vi "REWORK_config_keys_to_cluster.vi"(8 "error_in":errorcluster, 9 "section_key_type_table":string[][](array[string]), 10 "reference_ini_file_path":path, 11 "config_cluster_ref":refnum<vi>) -> (0 "error_out":errorcluster, 3 "reference_info":T1)   [LabVIEW 2019]
uses:
  typedef/REWORK_config_info.ctl
  _misc/ini/config_info.ctl
  _misc/AULocalize/SubVIs/Get Localized Phrase Compact Interface 0D.vi
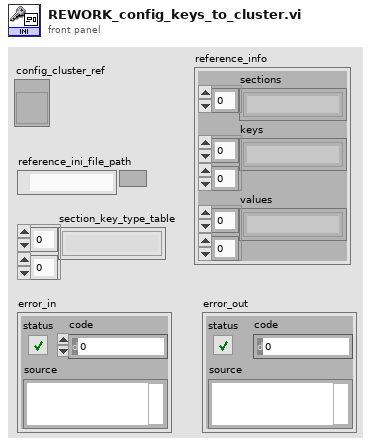
[diagram p1: front panel]
types:
  T1 = typedef "REWORK_config_info.ctl" = cluster{"sections":string[], "keys":string[][], "values":string[][]}
  T2 = typedef "config_info.ctl" = cluster{"sections":string[], "keys":string[][], "values":string[][]}
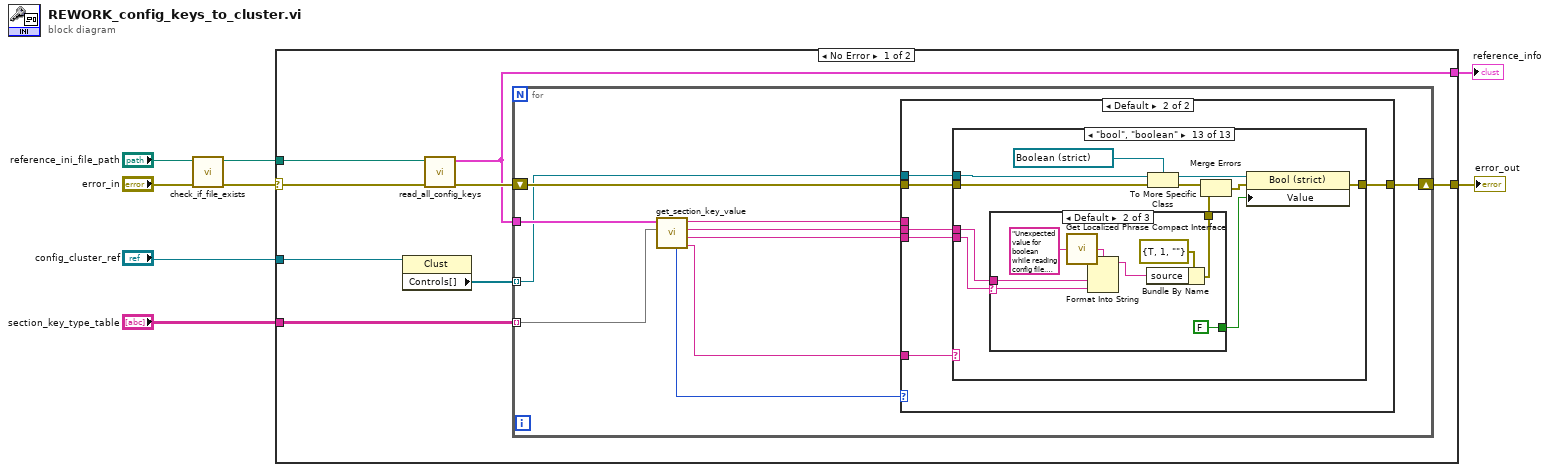
[diagram p0: block diagram]
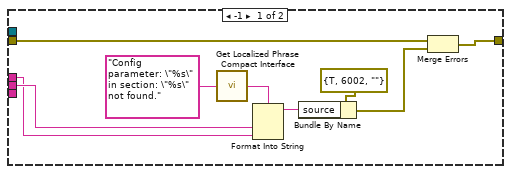
[diagram p2: hidden frame]
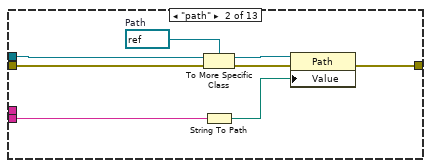
[diagram p4: hidden frame]
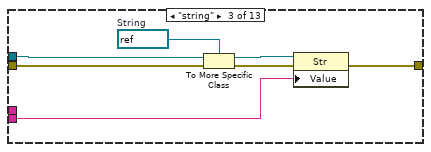
[diagram p5: hidden frame]
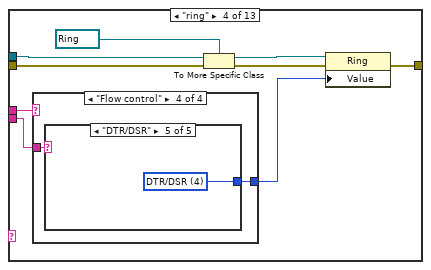
[diagram p6: hidden frame]
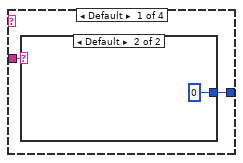
[diagram p7: hidden frame]
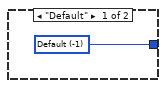
[diagram p8: hidden frame]
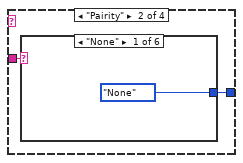
[diagram p9: hidden frame]
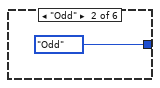
[diagram p10: hidden frame]
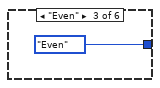
[diagram p11: hidden frame]
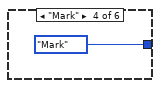
[diagram p12: hidden frame]
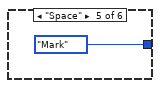
[diagram p13: hidden frame]
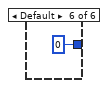
[diagram p14: hidden frame]
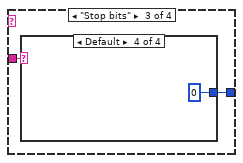
[diagram p15: hidden frame]
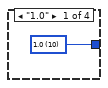
[diagram p16: hidden frame]
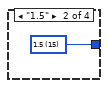
[diagram p17: hidden frame]
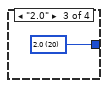
[diagram p18: hidden frame]
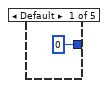
[diagram p19: hidden frame]
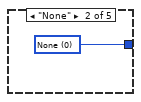
[diagram p20: hidden frame]
diagram:
  n1 = call "check_if_file_exists.vi"("error_in"="error_in", "file_path_in"="reference_ini_file_path") -> ("error_out"=w3:errorcluster, "file_path_out"=w2:path)  [unwired: 8 in]
  n2 = case shown="No Error" w3 {
    selector: w3 -> [w10 w208]
    tunnel: "section_key_type_table" -> [w16 _]
    tunnel: [w13 w208] -> w8
    tunnel: "config_cluster_ref" -> [w12 _]
    tunnel: [w11 T2 {"sections"=[], "keys"=[], "values"=[]} ("config_info")] -> w5
    tunnel: w2 -> [w9 _]
    frame No Error {
      n3 = property on="Property Node" class="Clust"(reference=w12) -> ("Controls[]"=w14:refnum<vi>[])  [unwired: 1 in, 2 out]
      n4 = call "read_all_config_keys.vi"("error_in"=w10, "config_file_path"=w9) -> ("error_out"=w15:errorcluster, "config_info"=w11:T2)  [unwired: 8 in]
      n5 = for {
        tunnel: w16 -> [w25] mode=indexing
        tunnel: w11 -> [w26]
        tunnel: w14 -> [w23] mode=indexing
        shift-right: [w22] -> w13
        shift-left: w15 -> [w24]
        n6 = call "get_section_key_value.vi"("section_key_type_table"=w25, "config_info"=w26) -> ("type"=w20:string, "value"=w19:string, "key"=w18:string, "section"=w17:string, "index of element"=w21:i32)  [unwired: 5 in]
        n7 = case shown="Default" w21 {
          tunnel: w19 -> [_ w41]
          tunnel: w20 -> [_ w40]
          tunnel: w24 -> [w34 w39]
          tunnel: w23 -> [_ w38]
          tunnel: [w35 w37] -> w22
          tunnel: w18 -> [w29 w36]
          tunnel: w17 -> [w28 _]
          frame -1 {
            n8 = call-poly "Get Localized Phrase Compact Interface.vi"("Key"="Config parameter: \"%s\" in section: \"%s\" not found." ("format string")) -> ("Translated Phrase"=w27:string)
            n9 = Format Into String(format string=w27, w29, w28) -> (resulting string=w31:string)  [unwired: 2 in, 1 out]
            n10 = Bundle By Name(cluster=errorcluster {"status"=TRUE, "code"=6002, "source"=""} ("error_out"), "source"=w31) -> (w32:errorcluster)
            n11 = Merge Errors(w34, w32) -> (w35:errorcluster)
          }
          frame Default {
            n12 = case shown="\"bool\", \"boolean\"" w40 {
              tunnel: w39 -> [w42 w50 w57 w66 w100 w134 w143 w152 w161 w170 w179 w185 w196]
              tunnel: w41 -> [_ w44 w52 w62 w96 w128 w136 w145 w154 w163 w172 w181 w192]
              tunnel: [w42 w43 w51 w63 w97 w130 w139 w148 w157 w166 w175 w183 w195] -> w37
              tunnel: w38 -> [_ w48 w55 w65 w99 w132 w141 w150 w159 w168 w177 w184 w190]
              tunnel: w36 -> [_ _ _ w58 w92 _ _ _ _ _ _ _ w186]
              frame Default {
              }
              frame "path" {
                w46 = refnum<vi> refnum  # Path
                n13 = To More Specific Class(target class=w46, reference=w48, error in=w50) -> (specific class reference=w47:refnum<vi>, error out=w49:errorcluster)
                n14 = String To Path(string=w44) -> (path=w45:path)
                n15 = property class="Path"(reference=w47, error in=w49, "Value"=w45) -> (error out=w43:errorcluster)  [unwired: 1 out]
              }
              frame "string" {
                w53 = refnum<vi> refnum  # String
                n16 = To More Specific Class(target class=w53, reference=w55, error in=w57) -> (specific class reference=w54:refnum<vi>, error out=w56:errorcluster)
                n17 = property class="Str"(reference=w54, error in=w56, "Value"=w52) -> (error out=w51:errorcluster)  [unwired: 1 out]
              }
              frame "ring" {
                n18 = case shown="\"Flow control\"" w58 {
                  tunnel: w62 -> [w68 w72 w80 w86]
                  tunnel: [w67 w71 w79 w85] -> w59
                  frame Default {
                    n19 = case shown="Default" w68 {
                      tunnel: [w69 0 ("input terminal configuration")] -> w67
                      frame "Default" {
                        w69 = -1 items=["Default"=-1, "RSE"=10083, "NRSE"=10078, "Differential"=10106, "Pseudodifferential"=12529] ("input terminal configuration")
                      }
                      frame Default {
                      }
                    }
                  }
                  frame "Pairity" {
                    n20 = case shown="\"None\"" w72 {
                      tunnel: [enum16{"None", "Odd", "Even", "Mark", "Space"}."None" ("SCANNER parity") enum16{"None", "Odd", "Even", "Mark", "Space"}."Odd" ("SCANNER parity") enum16{"None", "Odd", "Even", "Mark", "Space"}."Even" ("SCANNER parity") enum16{"None", "Odd", "Even", "Mark", "Space"}."Mark" ("SCANNER parity") enum16{"None", "Odd", "Even", "Mark", "Space"}."Mark" ("SCANNER parity") 0 ("input terminal configuration")] -> w71
                      frame "None" {
                      }
                      frame "Odd" {
                      }
                      frame "Even" {
                      }
                      frame "Mark" {
                      }
                      frame "Space" {
                      }
                      frame Default {
                      }
                    }
                  }
                  frame "Stop bits" {
                    n21 = case shown="Default" w80 {
                      tunnel: [w81 w82 w83 0 ("input terminal configuration")] -> w79
                      frame "1.0" {
                        w81 = u16 10 items=["1.0"=10, "1.5"=15, "2.0"=20] ("SCANNER stop bits")
                      }
                      frame "1.5" {
                        w82 = u16 15 items=["1.0"=10, "1.5"=15, "2.0"=20] ("SCANNER stop bits")
                      }
                      frame "2.0" {
                        w83 = u16 20 items=["1.0"=10, "1.5"=15, "2.0"=20] ("SCANNER stop bits")
                      }
                      frame Default {
                      }
                    }
                  }
                  frame "Flow control" {
                    n22 = case shown="\"DTR/DSR\"" w86 {
                      tunnel: [0 ("input terminal configuration") w88 w89 w90 w91] -> w85
                      frame Default {
                      }
                      frame "None" {
                        w88 = u16 0 items=["None"=0, "XON/XOFF"=1, "RTS/CTS"=2, "DTR/DSR"=4] ("SCANNER flow control")
                      }
                      frame "XON/XOFF" {
                        w89 = u16 1 items=["None"=0, "XON/XOFF"=1, "RTS/CTS"=2, "DTR/DSR"=4] ("SCANNER flow control")
                      }
                      frame "RTS/CTS" {
                        w90 = u16 2 items=["None"=0, "XON/XOFF"=1, "RTS/CTS"=2, "DTR/DSR"=4] ("SCANNER flow control")
                      }
                      frame "DTR/DSR" {
                        w91 = u16 4 items=["None"=0, "XON/XOFF"=1, "RTS/CTS"=2, "DTR/DSR"=4] ("SCANNER flow control")
                      }
                    }
                  }
                }
                n23 = To More Specific Class(target class=refnum<vi> refnum ("reference"), reference=w65, error in=w66) -> (specific class reference=w64:refnum<vi>, error out=w61:errorcluster)
                n24 = property class="Ring"(reference=w64, error in=w61, "Value"=w59) -> (error out=w63:errorcluster)  [unwired: 1 out]
              }
              frame "enum" {
                n25 = case shown="\"Flow control\"" w92 {
                  tunnel: w96 -> [w102 w106 w114 w120]
                  tunnel: [w101 w105 w113 w119] -> w93
                  frame Default {
                    n26 = case shown="Default" w102 {
                      tunnel: [w103 0 ("input terminal configuration")] -> w101
                      frame "Default" {
                        w103 = -1 items=["Default"=-1, "RSE"=10083, "NRSE"=10078, "Differential"=10106, "Pseudodifferential"=12529] ("input terminal configuration")
                      }
                      frame Default {
                      }
                    }
                  }
                  frame "Pairity" {
                    n27 = case shown="\"None\"" w106 {
                      tunnel: [enum16{"None", "Odd", "Even", "Mark", "Space"}."None" ("SCANNER parity") enum16{"None", "Odd", "Even", "Mark", "Space"}."Odd" ("SCANNER parity") enum16{"None", "Odd", "Even", "Mark", "Space"}."Even" ("SCANNER parity") enum16{"None", "Odd", "Even", "Mark", "Space"}."Mark" ("SCANNER parity") enum16{"None", "Odd", "Even", "Mark", "Space"}."Mark" ("SCANNER parity") 0 ("input terminal configuration")] -> w105
                      frame "None" {
                      }
                      frame "Odd" {
                      }
                      frame "Even" {
                      }
                      frame "Mark" {
                      }
                      frame "Space" {
                      }
                      frame Default {
                      }
                    }
                  }
                  frame "Stop bits" {
                    n28 = case shown="Default" w114 {
                      tunnel: [w115 w116 w117 0 ("input terminal configuration")] -> w113
                      frame "1.0" {
                        w115 = u16 10 items=["1.0"=10, "1.5"=15, "2.0"=20] ("SCANNER stop bits")
                      }
                      frame "1.5" {
                        w116 = u16 15 items=["1.0"=10, "1.5"=15, "2.0"=20] ("SCANNER stop bits")
                      }
                      frame "2.0" {
                        w117 = u16 20 items=["1.0"=10, "1.5"=15, "2.0"=20] ("SCANNER stop bits")
                      }
                      frame Default {
                      }
                    }
                  }
                  frame "Flow control" {
                    n29 = case shown="\"DTR/DSR\"" w120 {
                      tunnel: [0 ("input terminal configuration") w122 w123 w124 w125] -> w119
                      frame Default {
                      }
                      frame "None" {
                        w122 = u16 0 items=["None"=0, "XON/XOFF"=1, "RTS/CTS"=2, "DTR/DSR"=4] ("SCANNER flow control")
                      }
                      frame "XON/XOFF" {
                        w123 = u16 1 items=["None"=0, "XON/XOFF"=1, "RTS/CTS"=2, "DTR/DSR"=4] ("SCANNER flow control")
                      }
                      frame "RTS/CTS" {
                        w124 = u16 2 items=["None"=0, "XON/XOFF"=1, "RTS/CTS"=2, "DTR/DSR"=4] ("SCANNER flow control")
                      }
                      frame "DTR/DSR" {
                        w125 = u16 4 items=["None"=0, "XON/XOFF"=1, "RTS/CTS"=2, "DTR/DSR"=4] ("SCANNER flow control")
                      }
                    }
                  }
                }
                n30 = To More Specific Class(target class=refnum<vi> refnum ("reference"), reference=w99, error in=w100) -> (specific class reference=w98:refnum<vi>, error out=w95:errorcluster)
                n31 = property class="Enum"(reference=w98, error in=w95, "Value"=w93) -> (error out=w97:errorcluster)  [unwired: 1 out]
              }
              frame "U8" {
                w129 = u8 0  # U8
                n32 = Decimal String To Number(string=w128, default (0L)=w129) -> (number=w126:u8)  [unwired: 1 in, 1 out]
                n33 = To More Specific Class(target class=refnum<vi> refnum ("reference"), reference=w132, error in=w134) -> (specific class reference=w131:refnum<vi>, error out=w133:errorcluster)
                n34 = property class="Num"(reference=w131, error in=w133, "Value"=w126) -> (error out=w130:errorcluster)  [unwired: 1 out]
              }
              frame "U16" {
                w135 = refnum<vi> refnum  # Numeric
                w137 = u16 0  # U16
                n35 = Decimal String To Number(string=w136, default (0L)=w137) -> (number=w138:u16)  [unwired: 1 in, 1 out]
                n36 = To More Specific Class(target class=w135, reference=w141, error in=w143) -> (specific class reference=w140:refnum<vi>, error out=w142:errorcluster)
                n37 = property class="Num"(reference=w140, error in=w142, "Value"=w138) -> (error out=w139:errorcluster)  [unwired: 1 out]
              }
              frame "U32" {
                w146 = u32 0  # U32
                n38 = Decimal String To Number(string=w145, default (0L)=w146) -> (number=w147:u32)  [unwired: 1 in, 1 out]
                n39 = To More Specific Class(target class=refnum<vi> refnum ("reference"), reference=w150, error in=w152) -> (specific class reference=w149:refnum<vi>, error out=w151:errorcluster)
                n40 = property class="Num"(reference=w149, error in=w151, "Value"=w147) -> (error out=w148:errorcluster)  [unwired: 1 out]
              }
              frame "I8" {
                w155 = i8 0  # I8
                n41 = Decimal String To Number(string=w154, default (0L)=w155) -> (number=w156:i8)  [unwired: 1 in, 1 out]
                n42 = To More Specific Class(target class=refnum<vi> refnum ("reference"), reference=w159, error in=w161) -> (specific class reference=w158:refnum<vi>, error out=w160:errorcluster)
                n43 = property class="Num"(reference=w158, error in=w160, "Value"=w156) -> (error out=w157:errorcluster)  [unwired: 1 out]
              }
              frame "I16" {
                w164 = i16 0  # I16
                n44 = Decimal String To Number(string=w163, default (0L)=w164) -> (number=w165:i16)  [unwired: 1 in, 1 out]
                n45 = To More Specific Class(target class=refnum<vi> refnum ("reference"), reference=w168, error in=w170) -> (specific class reference=w167:refnum<vi>, error out=w169:errorcluster)
                n46 = property class="Num"(reference=w167, error in=w169, "Value"=w165) -> (error out=w166:errorcluster)  [unwired: 1 out]
              }
              frame "I32" {
                w173 = 0  # I32
                n47 = Decimal String To Number(string=w172, default (0L)=w173) -> (number=w174:i32)  [unwired: 1 in, 1 out]
                n48 = To More Specific Class(target class=refnum<vi> refnum ("reference"), reference=w177, error in=w179) -> (specific class reference=w176:refnum<vi>, error out=w178:errorcluster)
                n49 = property class="Num"(reference=w176, error in=w178, "Value"=w174) -> (error out=w175:errorcluster)  [unwired: 1 out]
              }
              frame "double", "real" {
                n50 = Fract/Exp String To Number(use system decimal point (T)=FALSE, string=w181) -> (number=w182:dbl)  [unwired: 2 in, 1 out]
                n51 = property class="Ctl"(reference=w184, error in=w185, "Value"=w182) -> (error out=w183:errorcluster)  [unwired: 1 out]
              }
              frame "bool", "boolean" {
                n52 = case shown="Default" w192 {
                  selector: w192 -> [_ w200 _]
                  tunnel: [FALSE FALSE TRUE] -> w191
                  tunnel: [_ w203 _] -> w187
                  tunnel: w186 -> [_ w199 _]
                  frame "0", "FALSE", "NO" {
                  }
                  frame Default {
                    n53 = call-poly "Get Localized Phrase Compact Interface.vi"("Key"="Unexpected value for boolean while reading config file. Following value is incorrect:\nParameter: %s\nValue: %s" ("source")) -> ("Translated Phrase"=w198:string)
                    n54 = Format Into String(format string=w198, w199, w200) -> (resulting string=w201:string)  [unwired: 2 in, 1 out]
                    n55 = Bundle By Name(cluster=errorcluster {"status"=TRUE, "code"=1, "source"=""} ("error constant"), "source"=w201) -> (w203:errorcluster)
                  }
                  frame "1", "TRUE", "YES" {
                  }
                }
                n56 = To More Specific Class(target class=refnum<vi> refnum ("reference"), reference=w190, error in=w196) -> (specific class reference=w194:refnum<vi>, error out=w189:errorcluster)
                n57 = Merge Errors(w189, w187) -> (w188:errorcluster)
                n58 = property class="Bool (strict)"(reference=w194, error in=w188, "Value"=w191) -> (error out=w195:errorcluster)  [unwired: 1 out]
              }
            }
          }
        }
      }
    }
    frame Error {
    }
  }
  "error_out" <- w8
  "reference_info" <- w5
